vi "SensorInterface_UserEventShutdown.vi"(7 "Action":T1, 8 "error in (no error)":errorcluster) -> (0 "error out":errorcluster, 3 "Ref out":refnum<user-event>)   [LabVIEW 2013]
doc: "This VI handles SensorI nterface loop shutdowns service. \n\nThis is Functional Global Variable."
uses:
  General/Controls/#TD_General_UserEventStates_Enum.ctl
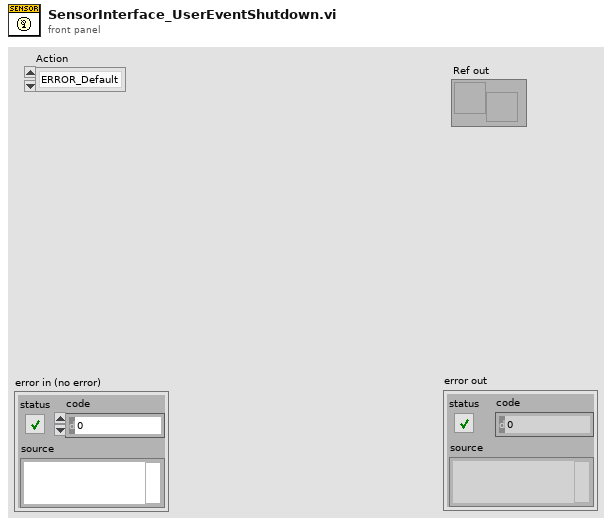
[diagram p1: front panel]
types:
  T1 = typedef "#TD_General_UserEventStates_Enum.ctl" = enum16{"ERROR_Default", "Create", "GetRef", "Generate", "Release"}
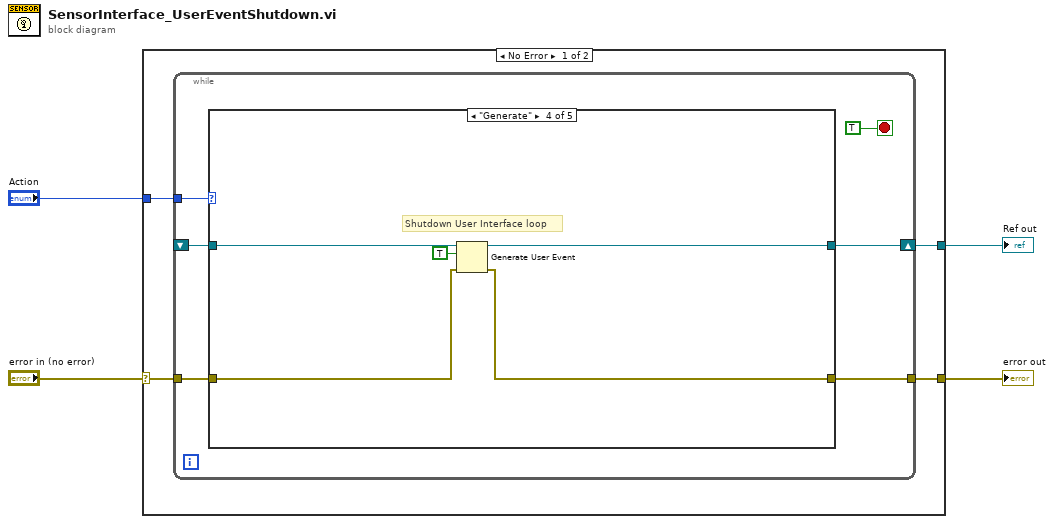
[diagram p0: block diagram]
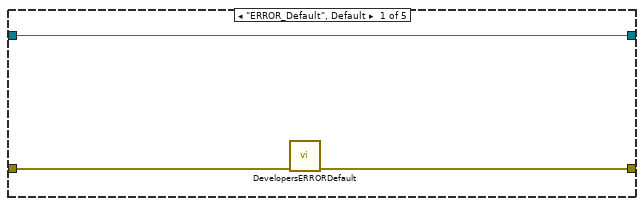
[diagram p2: hidden frame]
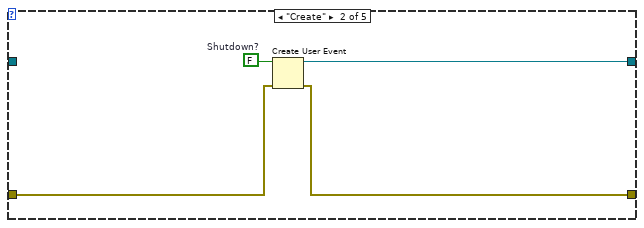
[diagram p3: hidden frame]
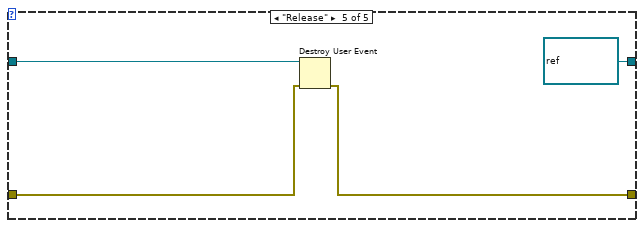
[diagram p5: hidden frame]
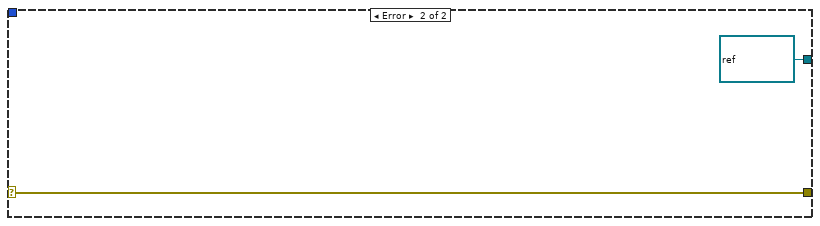
[diagram p6: hidden frame]
diagram:
  n1 = case shown="No Error" "error in (no error)" {
    selector: "error in (no error)" -> [w7 w33]
    tunnel: "Action" -> [w8 _]
    tunnel: [w6 refnum<user-event> refnum ("Shutdown?")] -> w1
    tunnel: [w5 w33] -> w2
    frame No Error {
      n2 = while {
        tunnel: w8 -> [w14]
        tunnel: w7 -> [w13]
        tunnel: [w11] -> w5
        shift-right: [w12] -> w6
        shift-left: _ -> [w9]
        stop <- TRUE stop-if-true
        n3 = case shown="\"Generate\"" w14 {
          tunnel: w13 -> [w16 w21 w22 w27 w31]
          tunnel: [w15 w19 w23 w24 refnum<user-event> refnum ("Shutdown?")] -> w12
          tunnel: [w17 w18 w22 w26 w30] -> w11
          tunnel: w9 -> [w15 _ w23 w28 w32]
          frame "ERROR_Default", Default {
            n4 = call "DevelopersERRORDefault.vi"("error in (no error)"=w16) -> ("error out"=w17:errorcluster)  [unwired: 10 in]
          }
          frame "Create" {
            w20 = FALSE  # Shutdown?
            n5 = Create User Event(user event datatype=w20, error in=w21) -> (user event=w19:refnum<user-event>, error out=w18:errorcluster)
          }
          frame "GetRef" {
          }
          frame "Generate" {
            # "Shutdown User Interface loop"
            n6 = Generate User Event(user event=w28, event data cluster=TRUE ("event data"), error in=w27) -> (user event out=w24:refnum<user-event>, error out=w26:errorcluster)  [unwired: 1 in]
          }
          frame "Release" {
            n7 = Destroy User Event(user event=w32, error in=w31) -> (error out=w30:errorcluster)
          }
        }
      }
    }
    frame Error {
    }
  }
  "error out" <- w2
  "Ref out" <- w1
